vi "Conv_JSON_1 (SubVI).vi"(9 "data":string[](array[string]), 11 "Cluster":T1) -> (1 "payload length":i32, 3 "String":string)   [LabVIEW 2015]
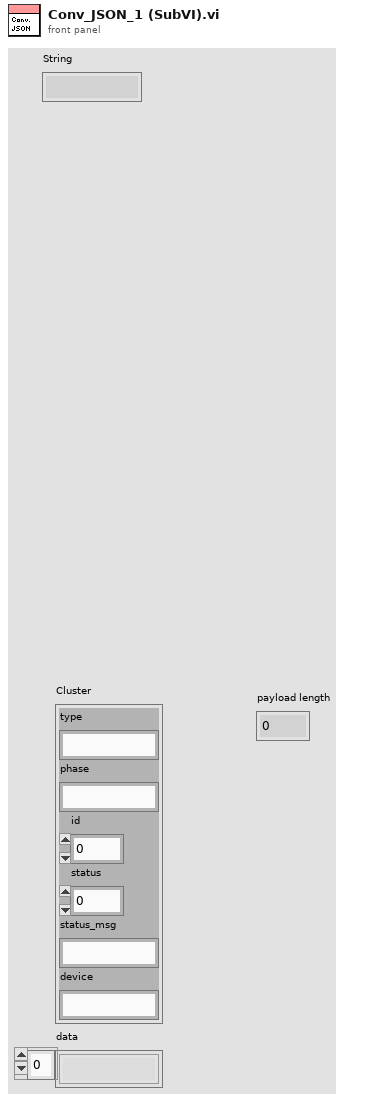
[diagram p1: front panel]
types:
  T1 = cluster{"type":string, "phase":string, "id":u8, "status":i32, "status_msg":string, "device":string}
  T2 = cluster{"type":string, "phase":string, "id":u8, "status":i32, "status_msg":string, "device":string, "data":string[]}
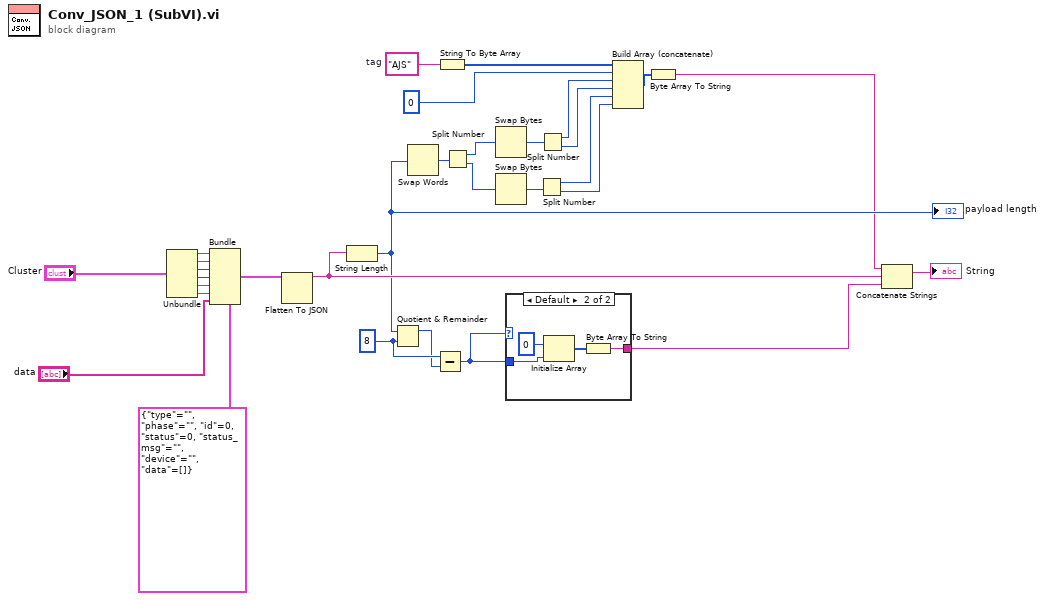
[diagram p0: block diagram]
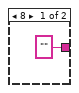
[diagram p2: hidden frame]
diagram:
  w29 = 8 ("y")
  w24 = "AJS"  # tag
  n1 = Unbundle("Cluster") -> ("type"=w13:string, "phase"=w12:string, "id"=w11:u8, "status"=w10:i32, "status_msg"=w9:string, "device"=w8:string)
  n2 = Bundle(cluster=T2 {"type"="", "phase"="", "id"=0, "status"=0, "status_msg"="", "device"="", "data"=[]}, "type"=w13, "phase"=w12, "id"=w11, "status"=w10, "status_msg"=w9, "device"=w8, "data"="data") -> (w6:T2)
  n3 = Flatten To JSON(anything=w6) -> (JSON string=w30:string)  [unwired: 2 in, 1 out]
  n4 = String Length(string=w30) -> (length=w28:i32)
  "payload length" <- w28
  n5 = Quotient & Remainder(x=w28, y=w29) -> (x-y*floor(x/y)=w3:i32)  [unwired: 1 out]
  n6 = Swap Words(1:w28) -> (0:w27:i32)
  n7 = Subtract(x=w29, y=w3) -> (x-y=w1:i32)
  n8 = String To Byte Array(string=w24) -> (unsigned byte array=w23:u8[])
  n9 = Split Number(x=w27) -> (hi(x)=w26:u16, lo(x)=w25:u16)
  n10 = Swap Bytes(anything=w26) -> (byte swapped=w18:u16)
  n11 = Swap Bytes(anything=w25) -> (byte swapped=w19:u16)
  n12 = case shown="Default" w1 {
    tunnel: ["" ("string") w34] -> w2
    tunnel: w1 -> [_ w33]
    frame 8 {
    }
    frame Default {
      n13 = Initialize Array(u8 0 ("element"), w33) -> (w35:u8[])
      n14 = Byte Array To String(unsigned byte array=w35) -> (string=w34:string)
    }
  }
  n15 = Split Number(x=w19) -> (hi(x)=w15:u8, lo(x)=w14:u8)
  n16 = Split Number(x=w18) -> (hi(x)=w17:u8, lo(x)=w16:u8)
  n17 = Build Array (concatenate)(w23, u8 0, w17, w16, w15, w14) -> (w21:u8[])
  n18 = Byte Array To String(unsigned byte array=w21) -> (string=w20:string)
  n19 = Concatenate Strings(w20, w30, w2) -> (→"String":string)
